vi "_024.vi"() -> ()   [LabVIEW 2024]
panel:
  out "Boolean 2":bool=TRUE
  in  "stop 2":bool
  out "Waveform Chart 2":dbl(graph)
  out "Indicator":bool=TRUE
  out "Waveform Chart":dbl(graph)
  in  "stop":bool
  # "Flat Sequence Structure :"
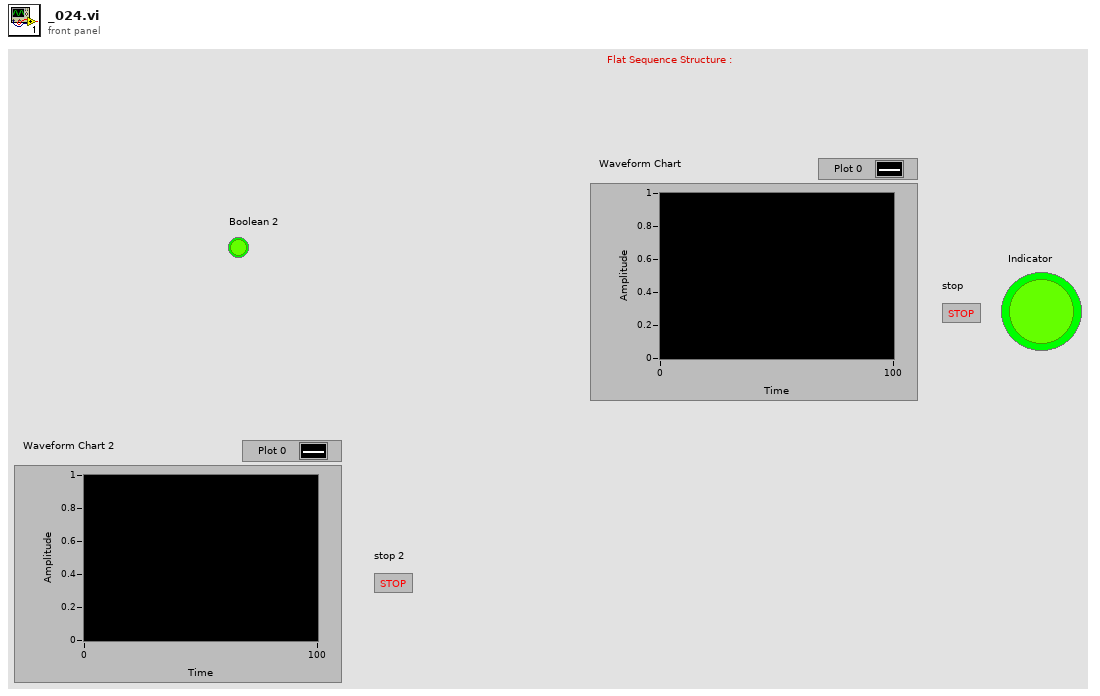
[diagram p1: front panel]
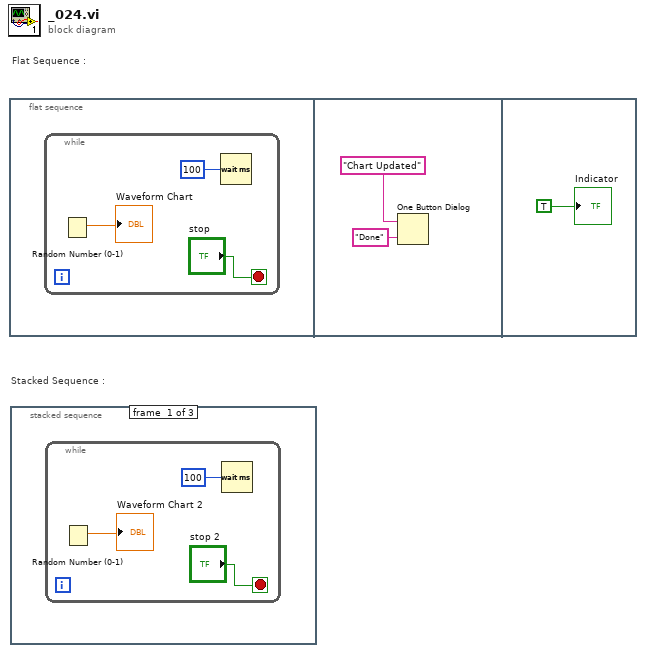
[diagram p0: block diagram]
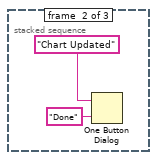
[diagram p2: hidden frame]
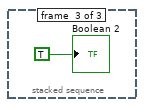
[diagram p3: hidden frame]
diagram:
  # "Flat Sequence :"
  # "Stacked Sequence :"
  n1 = flat-sequence {
    frame #0 {
      n2 = while {
        stop <- "stop" stop-if-true
        n3 = Random Number (0-1)() -> (number: 0 to 1=→"Waveform Chart":dbl)
        n4 = Wait (ms)(milliseconds to wait=u32 100 ("millisecond timer value")) -> ()  [unwired: 1 out]
      }
    }
    frame #1 {
      n5 = One Button Dialog(message="Chart Updated", button name ("OK")="Done") -> ()  [unwired: 1 out]
    }
    frame #2 {
      "Indicator" <- TRUE
    }
  }
  n6 = stacked-sequence {
    frame #0 {
      n7 = while {
        stop <- "stop 2" stop-if-true
        n8 = Random Number (0-1)() -> (number: 0 to 1=→"Waveform Chart 2":dbl)
        n9 = Wait (ms)(milliseconds to wait=u32 100 ("millisecond timer value")) -> ()  [unwired: 1 out]
      }
    }
    frame #1 {
      n10 = One Button Dialog(message="Chart Updated", button name ("OK")="Done") -> ()  [unwired: 1 out]
    }
    frame #2 {
      "Boolean 2" <- TRUE
    }
  }
